vi "Get Function.vi"(8 "error in (no error)":errorcluster, 11 "measurement_type":string) -> (0 "error out":errorcluster, 3 "function":u16(ring) items=["DC Voltage", "AC Voltage", "2 - Wire Resistance", "4 - Wire Resistance", "DC Current", "AC Current", "Frequency", "Period", "Continuity", "Diode Checking", "VDC:VDC Ratio", "Temperature", "Capacitance"])   [LabVIEW 2020, in "Keysight 34401A DMM Measurement.lvlib"]
uses:
  Keysight 34401A DMM Measurement.lvlib
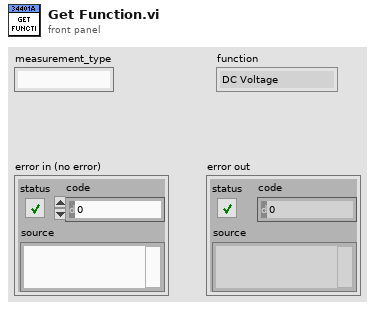
[diagram p1: front panel]
types:
  T1 = cluster{string, "Function (0: DC Voltage)":u16}[]
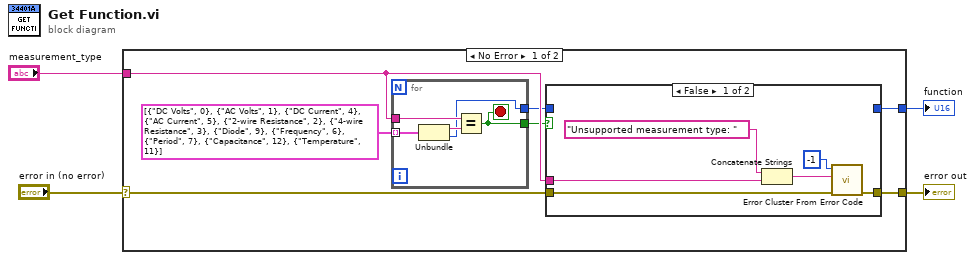
[diagram p0: block diagram]
diagram:
  n1 = case shown="No Error" "error in (no error)" {
    selector: "error in (no error)" -> [w6 w25]
    tunnel: [w11 w25] -> w4
    tunnel: "measurement_type" -> [w10 _]
    tunnel: [w8 _] -> w1
    frame No Error {
      n2 = for {
        tunnel: T1 [{"DC Volts", "Function (0: DC Voltage)"=0}, {"AC Volts", "Function (0: DC Voltage)"=1}, {"DC Current", "Function (0: DC Voltage)"=4}, {"AC Current", "Function (0: DC Voltage)"=5}, {"2-wire Resistance", "Function (0: DC Voltage)"=2}, {"4-wire Resistance", "Function (0: DC Voltage)"=3}, {"Diode", "Function (0: DC Voltage)"=9}, {"Frequency", "Function (0: DC Voltage)"=6}, {"Period", "Function (0: DC Voltage)"=7}, {"Capacitance", "Function (0: DC Voltage)"=12}, {"Temperature", "Function (0: DC Voltage)"=11}] -> [w24] mode=indexing
        tunnel: w10 -> [w22]
        tunnel: [w21] -> w7
        tunnel: [w20] -> w9
        stop <- w20 stop-if-true
        n3 = Unbundle(w24) -> (w23:string, "Function (0: DC Voltage)"=w21:u16)
        n4 = Equal?(x=w22, y=w23) -> (x = y?=w20:bool)
      }
      n5 = case shown="False" w9 {
        tunnel: w6 -> [w17 w18]
        tunnel: [w16 w18] -> w11
        tunnel: w10 -> [w13 _]
        tunnel: [_ w19] -> w8
        tunnel: w7 -> [_ w19]
        frame False {
          n6 = Concatenate Strings("Unsupported measurement type: ", w13) -> (w12:string)
          n7 = call <vilib>:"Error Cluster From Error Code.vi"("error in (no error)"=w17, "error message (\"\")"=w12, "error code (0)"=-1) -> ("error out"=w16:errorcluster)  [unwired: 6 in]
        }
        frame True {
        }
      }
    }
    frame Error {
    }
  }
  "error out" <- w4
  "function" <- w1
